vi "Station Retrieve Record.vi"(8 "error in (no error)":errorcluster, 11 "Statement Refnum":T1) -> (0 "error out":errorcluster, 2 "Station Record":T2, 3 "Statement Refnum":T1)   [LabVIEW 2011]
uses:
  Station Record.ctl
  Summitek EXT/ODBC/SQL Controls/Statement Refnum.ctl
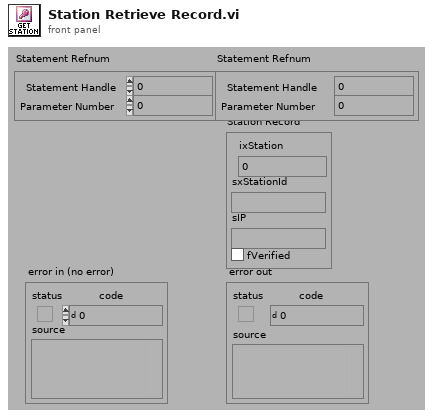
[diagram p1: front panel]
types:
  T1 = typedef "Statement Refnum.ctl" = cluster{"Statement Handle":i32, "Parameter Number":u16}
  T2 = typedef "Station Record.ctl" = cluster{"ixStation":i32, "sxStationId":string, "sIP":string, "fVerified":bool}
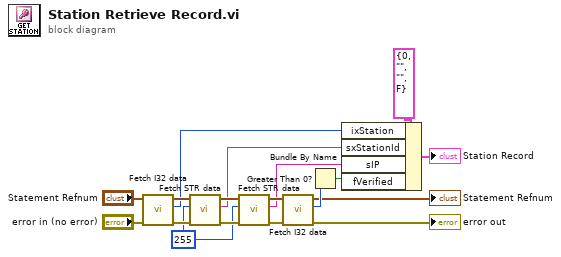
[diagram p0: block diagram]
diagram:
  w12 = 255 ("Buffer Size")
  n1 = call "Fetch I32 data.vi"("error in (no error)"="error in (no error)", "Statement Refnum"="Statement Refnum") -> ("error out"=w14:errorcluster, "Data"=w3:i32, "Statement Refnum"=w13:T1)  [unwired: 3 out]
  n2 = call "Fetch STR data.vi"("error in (no error)"=w14, "Buffer Size"=w12, "Statement Refnum"=w13) -> ("error out"=w16:errorcluster, "Data"=w4:string, "Statement Refnum"=w15:T1)  [unwired: 2 out]
  n3 = call "Fetch STR data.vi"("error in (no error)"=w16, "Buffer Size"=w12, "Statement Refnum"=w15) -> ("error out"=w8:errorcluster, "Data"=w5:string, "Statement Refnum"=w9:T1)  [unwired: 2 out]
  n4 = call "Fetch I32 data.vi"("error in (no error)"=w8, "Statement Refnum"=w9) -> ("error out"=→"error out":errorcluster, "Data"=w11:i32, "Statement Refnum"=→"Statement Refnum":T1)  [unwired: 3 out]
  n5 = Greater Than 0?(x=w11) -> (x > 0?=w7:bool)
  n6 = Bundle By Name(cluster=T2 {"ixStation"=0, "sxStationId"="", "sIP"="", "fVerified"=FALSE} ("Station Information"), "ixStation"=w3, "sxStationId"=w4, "sIP"=w5, "fVerified"=w7) -> (→"Station Record":T2)
